vi "子界面-查看某框和报告生成-第2版-不显示界面.vi"(0 "框号":dbl format="%#_13g", 1 "框组":T3(array[cluster]), 3 "反射图原始路径":path, 5 "预先配置的灰度阈值":dbl, 6 "穿透图原始路径":path, 7 "部位信息":string[](array[string])=["", "34.500000", "32.500000", "1121", "34", "54.955926", "分层类", "不合格", ""], 12 "产品规格":cluster{"产品长度（周长）（mm）":dbl, "产品宽度（母线长）（mm）":dbl}) -> (14 "弥散类检测结果":string[][](table), 19 "分层类检测结果":string[][](table))   [LabVIEW 2018]
uses:
  <vilib>/vision/NI_Vision_Development_Module.lvlib
panel:
  out "弥散缺陷个数":i32
  out "分层缺陷个数":i32
  out "合格？ 弥散类":string="fencengThreshold"
  out "合格？分层类":string="fencengThreshold"
  out "?":T1(plugin-control)
  out "Threshold Image":T1(plugin-control)
  out "Threshold Image":T1(plugin-control)
  out "Threshold Image":T1(plugin-control)
  out "反射图ROI的最大灰度值":sgl
  in  "灰度阈值设置":cluster{"下限":dbl, "下限":dbl}(slide)={"下限"=0.0, "下限"=65.10638427734375} scale=0.0..255.0
  in  "Tab Control":T2
  out "穿透ROI":T1(plugin-control)
  out "Threshold Image":T1(plugin-control)
  out "?":T1(plugin-control)
  out "?":T1(plugin-control)
  out "Threshold Image":T1(plugin-control)
  out "Threshold Image":T1(plugin-control)
  out "弥散测量结果":dbl[][](array[numeric]) format="%.2f"
  in  "分隔符（'\\'代码显示）":string="\t"
  in  "格式字符串":string="%f"
  out "面积 (pixels)":i32
  in  "格式字符串 2":string="%f"
  in  "分隔符（'\\'代码显示）":string="\t"
  out "分层测量结果":dbl[][](array[numeric]) format="%.2f"
  out "缺陷分类的临界值":sgl format="%#.3f"
  # "所选区域信息"
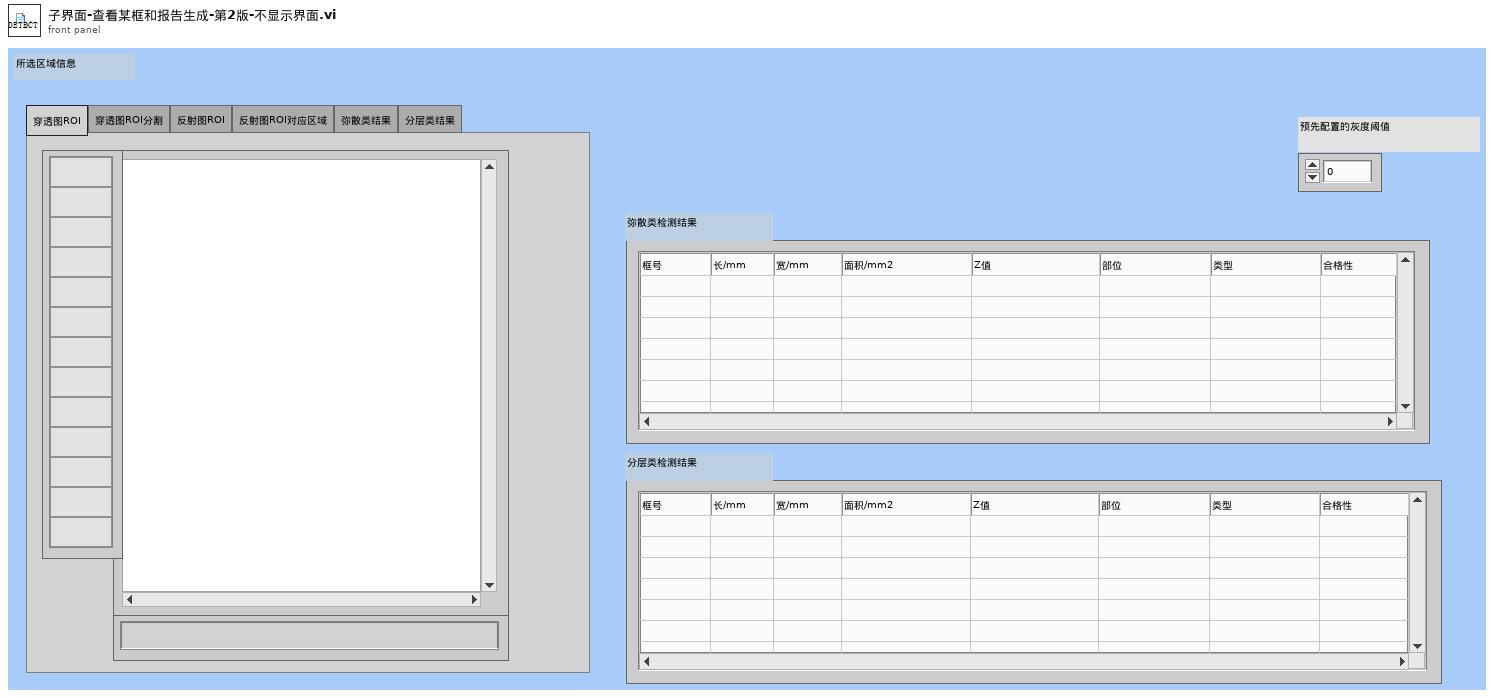
[diagram p1: front panel]
types:
  T1 = typedef "IMAQ Image.ctl" = refnum<image>
  T2 = typedef "控件 1.ctl" = enum32{"穿透图ROI", "穿透图ROI分割", "反射图ROI", "反射图ROI对应区域", "弥散类结果", "分层类结果"}
  T3 = cluster{"Global Rectangle":i32[], "Contours":cluster{"Contour Type":u32, "ROI Type":u32, "Points":i32[]}[]}[]
  T4 = typedef "Image Type" = u32
  T5 = typedef "Particle Parameters" = i32
  T6 = cluster{"Measurement Parameter":T5, "Range Lower Value":dbl, "Range Upper Value":dbl, "Range":bool, "Measurement Type":bool}[]
  T7 = cluster{"Global Rectangle":i32[], "Contours":cluster{"Contour Type":u32, "ROI Type":u32, "Points":i32[]}[]}
  T8 = cluster{"histogram":u32[], "Minimal Value":sgl, "Maximal Value":sgl, "Starting Value":sgl, "Interval Width":sgl, "Mean Value":sgl, "Standard  Variation":sgl, "Area (pixels)":i32}
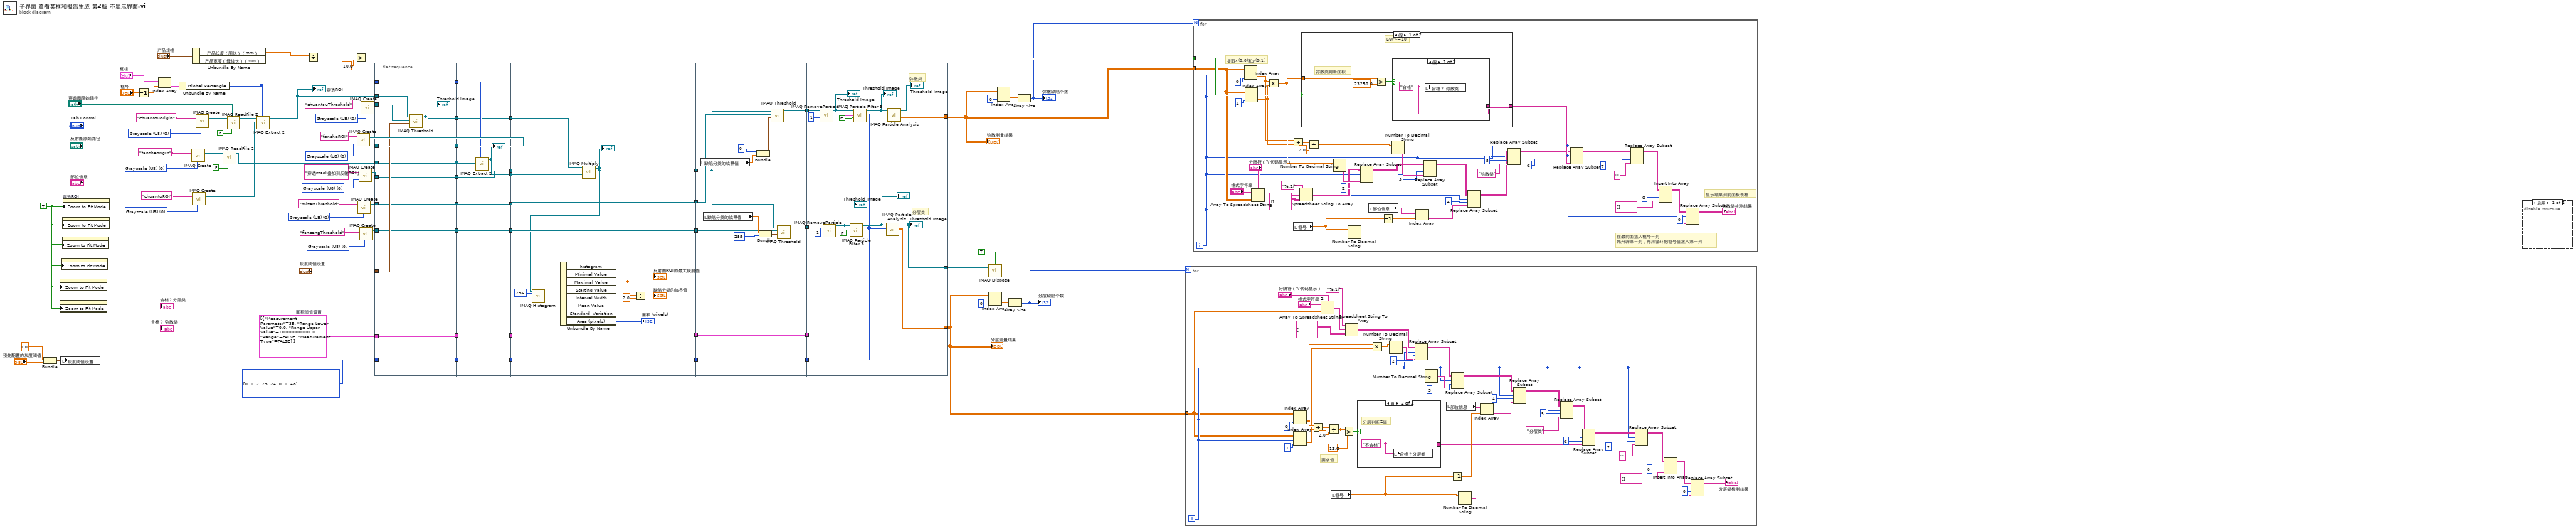
[diagram p0: block diagram]
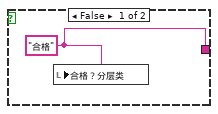
[diagram p2: hidden frame]
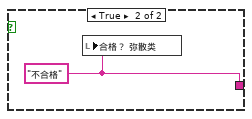
[diagram p3: hidden frame]
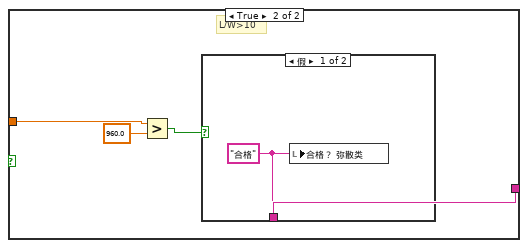
[diagram p4: hidden frame]
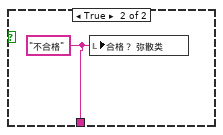
[diagram p5: hidden frame]
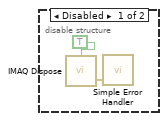
[diagram p6: hidden frame]
diagram:
  w48 = T4 0 items=["Grayscale (U8)", "Grayscale (I16)", "Grayscale (SGL)", "Complex (CSG)", "RGB (U32)", "HSL (U32)", "RGB (U64)", "Grayscale (U16)"] ("Image Type")
  w49 = T4 0 items=["Grayscale (U8)", "Grayscale (I16)", "Grayscale (SGL)", "Complex (CSG)", "RGB (U32)", "HSL (U32)", "RGB (U64)", "Grayscale (U16)"] ("Image Type")
  w50 = T4 0 items=["Grayscale (U8)", "Grayscale (I16)", "Grayscale (SGL)", "Complex (CSG)", "RGB (U32)", "HSL (U32)", "RGB (U64)", "Grayscale (U16)"] ("Image Type")
  w54 = T4 0 items=["Grayscale (U8)", "Grayscale (I16)", "Grayscale (SGL)", "Complex (CSG)", "RGB (U32)", "HSL (U32)", "RGB (U64)", "Grayscale (U16)"] ("Image Type")
  w58 = T4 0 items=["Grayscale (U8)", "Grayscale (I16)", "Grayscale (SGL)", "Complex (CSG)", "RGB (U32)", "HSL (U32)", "RGB (U64)", "Grayscale (U16)"] ("Image Type")
  w6 = i32[] [0, 1, 2, 23, 24, 0, 1, 48] items=["Bounding Rect Width", "Bounding Rect Height", "Area"] ("Pixel Measurements")
  w11 = T6 [{"Measurement Parameter"=35, "Range Lower Value"=0.0, "Range Upper Value"=10000000000.0, "Range"=FALSE, "Measurement Type"=FALSE}]  # 面积阈值设置
  w71 = T4 0 items=["Grayscale (U8)", "Grayscale (I16)", "Grayscale (SGL)", "Complex (CSG)", "RGB (U32)", "HSL (U32)", "RGB (U64)", "Grayscale (U16)"] ("Image Type")
  w41 = T4 0 items=["Grayscale (U8)", "Grayscale (I16)", "Grayscale (SGL)", "Complex (CSG)", "RGB (U32)", "HSL (U32)", "RGB (U64)", "Grayscale (U16)"] ("Image Type")
  w75 = T4 0 items=["Grayscale (U8)", "Grayscale (I16)", "Grayscale (SGL)", "Complex (CSG)", "RGB (U32)", "HSL (U32)", "RGB (U64)", "Grayscale (U16)"] ("Image Type")
  w84 = TRUE ("Zoom to Fit Mode")
  n1 = Bundle(0.0, "预先配置的灰度阈值"="预先配置的灰度阈值") -> (w82:cluster{dbl, "预先配置的灰度阈值":dbl})  [unwired: 1 in]
  n2 = property class="ImageControl"("Zoom to Fit Mode"=w84) -> ()  [unwired: 2 in, 2 out]
  n3 = property class="ImageControl"("Zoom to Fit Mode"=w84) -> ()  [unwired: 2 in, 2 out]
  n4 = local write "灰度阈值设置"(w82) -> ()
  n5 = property class="ImageControl"("Zoom to Fit Mode"=w84) -> ()  [unwired: 2 in, 2 out]
  n6 = property class="ImageControl"("Zoom to Fit Mode"=w84) -> ()  [unwired: 2 in, 2 out]
  n7 = property class="ImageControl"("Zoom to Fit Mode"=w84) -> ()  [unwired: 2 in, 2 out]
  n8 = property on="穿透ROI" class="ImageControl"("Zoom to Fit Mode"=w84) -> ()  [unwired: 2 in, 2 out]
  n9 = Decrement(x="框号") -> (x-1=w77:dbl)
  n10 = Index Array(array="框组", index=w77) -> (element=w78:T7)
  n11 = Unbundle By Name(w78) -> ("Global Rectangle"=w40:i32[])
  n12 = call "IMAQ Create"("Image Name"="fansheorigin", "Image Type"=w54) -> ("New Image"=w53:T1)  [unwired: 3 in, 1 out]
  n13 = call "IMAQ Create"("Image Name"="chuantuROI", "Image Type"=w58) -> ("New Image"=w57:T1)  [unwired: 3 in, 1 out]
  n14 = Unbundle By Name("产品规格") -> ("产品长度（周长）（mm）"=w66:dbl, "产品宽度（母线长）（mm）"=w65:dbl)
  n15 = call "IMAQ Create"("Image Name"="chuantouorigin", "Image Type"=w75) -> ("New Image"=w60:T1)  [unwired: 3 in, 1 out]
  n16 = call "IMAQ ReadFile 2"("Use File Path Image Type"=FALSE, "File Path"="反射图原始路径", "Image"=w53) -> ("Image Out"=w35:T1)  [unwired: 4 in, 4 out]
  n17 = call "IMAQ ReadFile 2"("Use File Path Image Type"=FALSE, "File Path"="穿透图原始路径", "Image"=w60) -> ("Image Out"=w61:T1)  [unwired: 4 in, 4 out]
  n18 = call "IMAQ Extract 2"("Optional Rectangle"=w40, "Image Dst"=w57, "Image Src"=w61) -> ("Image Dst Out"=w38:T1)  [unwired: 7 in, 1 out]
  "穿透ROI" <- w38
  n19 = Divide(x=w66, y=w65) -> (x/y=w69:dbl)
  n20 = Greater?(x=w69, y=10.0) -> (0:w64:bool)
  n21 = call "IMAQ Create"("Image Name"="fansheROI", "Image Type"=w41) -> ("New Image"=w36:T1)  [unwired: 3 in, 1 out]
  n22 = call "IMAQ Create"("Image Name"="misanThreshold", "Image Type"=w48) -> ("New Image"=w22:T1)  [unwired: 3 in, 1 out]
  n23 = call "IMAQ Create"("Image Name"="穿透mask叠加到反射ROI上", "Image Type"=w71) -> ("New Image"=w30:T1)  [unwired: 3 in, 1 out]
  n24 = call "IMAQ Create"("Image Name"="fencengThreshold", "Image Type"=w49) -> ("New Image"=w20:T1)  [unwired: 3 in, 1 out]
  n25 = call "IMAQ Create"("Image Name"="chuantouThreshold", "Image Type"=w50) -> ("New Image"=w39:T1)  [unwired: 3 in, 1 out]
  n26 = flat-sequence {
    tunnel: w40 -> [w96]
    tunnel: w39 -> [w95]
    tunnel: w38 -> [w94]
    tunnel: "灰度阈值设置" -> [w93]
    tunnel: w36 -> [w92]
    tunnel: w35 -> [w91]
    tunnel: [w96] -> w34
    tunnel: [w92] -> w33
    tunnel: [w91] -> w32
    tunnel: [w90] -> w31
    tunnel: w30 -> [w90]
    tunnel: [w89] -> w27
    tunnel: w22 -> [w88]
    tunnel: [w88] -> w24
    tunnel: [w87] -> w21
    tunnel: w20 -> [w87]
    tunnel: [w86] -> w12
    tunnel: w11 -> [w86]
    tunnel: [w85] -> w7
    tunnel: w6 -> [w85]
    tunnel: w34 -> [w106]
    tunnel: w33 -> [w104]
    tunnel: w32 -> [w105]
    tunnel: w31 -> [w103]
    tunnel: [w103] -> w29
    tunnel: [w102] -> w28
    tunnel: w27 -> [w102]
    tunnel: [w101] -> w26
    tunnel: w24 -> [w100]
    tunnel: [w100] -> w23
    tunnel: w21 -> [w99]
    tunnel: [w99] -> w19
    tunnel: w12 -> [w98]
    tunnel: [w98] -> w10
    tunnel: w7 -> [w97]
    tunnel: [w97] -> w5
    tunnel: w29 -> [w120]
    tunnel: w28 -> [w119]
    tunnel: w26 -> [w118]
    tunnel: [w117] -> w25
    tunnel: w23 -> [w117]
    tunnel: w19 -> [w116]
    tunnel: [w116] -> w18
    tunnel: [w109] -> w17
    tunnel: w10 -> [w108]
    tunnel: [w108] -> w9
    tunnel: w5 -> [w107]
    tunnel: [w107] -> w4
    tunnel: w25 -> [w128]
    tunnel: w18 -> [w127]
    tunnel: w17 -> [w126]
    tunnel: [w125] -> w14
    tunnel: [w124] -> w13
    tunnel: w9 -> [w123]
    tunnel: [w123] -> w8
    tunnel: w4 -> [w122]
    tunnel: [w122] -> w3
    tunnel: [w144] -> w16
    tunnel: [w139] -> w1
    tunnel: [w138] -> w15
    tunnel: w14 -> [w137]
    tunnel: w13 -> [w136]
    tunnel: w8 -> [w135]
    tunnel: w3 -> [w134]
    frame #0 {
      n27 = call "IMAQ Threshold"("Range"=w93, "Image Dst"=w95, "Image Src"=w94) -> ("Image Dst Out"=w89:T1)  [unwired: 3 in, 5 out]
      "Threshold Image" <- w89
    }
    frame #1 {
      n28 = call "IMAQ Extract 2"("Optional Rectangle"=w106, "Image Dst"=w105, "Image Src"=w104) -> ("Image Dst Out"=w101:T1)  [unwired: 7 in, 1 out]
      "?" <- w101
    }
    frame #2 {
      n29 = call "IMAQ Multiply"("Image Src A"=w119, "Image Dst"=w120, "Image Src B"=w118) -> ("Image Dst Out"=w109:T1)  [unwired: 4 in, 1 out]
      "?" <- w109
      n30 = call "IMAQ Histogram"("Number of Classes"=256, "Image"=w109) -> ("Histogram Report"=w112:T8)  [unwired: 8 in, 1 out]
      n31 = Unbundle By Name(w112) -> ("Maximal Value"=w114:sgl, "Area (pixels)"=→"面积 (pixels)":i32)  [unwired: 6 out]
      "反射图ROI的最大灰度值" <- w114
      n32 = Divide(x=w114, y=sgl 2.0) -> (x/y=→"缺陷分类的临界值":sgl)
    }
    frame #3 {
      n33 = local read "缺陷分类的临界值"() -> (w133:sgl)
      n34 = local read "缺陷分类的临界值"() -> (w131:sgl)
      n35 = Bundle(0, "缺陷分类的临界值"=w133) -> (w121:cluster{i32, "缺陷分类的临界值":sgl})  [unwired: 1 in]
      n36 = Bundle("缺陷分类的临界值"=w131, 255) -> (w130:cluster{"缺陷分类的临界值":sgl, i32})  [unwired: 1 in]
      n37 = call "IMAQ Threshold"("Range"=w121, "Image Dst"=w128, "Image Src"=w126) -> ("Image Dst Out"=w124:T1)  [unwired: 3 in, 5 out]
      n38 = call "IMAQ Threshold"("Range"=w130, "Image Dst"=w127, "Image Src"=w126) -> ("Image Dst Out"=w125:T1)  [unwired: 3 in, 5 out]
    }
    frame #4 {
      # "分层类"
      # "弥散类"
      n39 = call "IMAQ RemoveParticle"("Number of Erosion"=1, "Image Src"=w136) -> ("Image Dst Out"=w147:T1)  [unwired: 8 in, 1 out]
      "Threshold Image" <- w147
      n40 = call "IMAQ RemoveParticle"("Number of Erosion"=1, "Image Src"=w137) -> ("Image Dst Out"=w142:T1)  [unwired: 8 in, 1 out]
      "Threshold Image" <- w142
      n41 = call "IMAQ Particle Filter 3"("Image Src"=w142, "Keep/Remove Particles (F)"=FALSE) -> ("Image Dst Out"=w143:T1)  [unwired: 11 in, 2 out]
      "?" <- w143
      n42 = call "IMAQ Particle Filter 3"("Image Src"=w147, "Selection Values"=w135, "Keep/Remove Particles (F)"=FALSE) -> ("Image Dst Out"=w148:T1)  [unwired: 10 in, 2 out]
      "Threshold Image" <- w148
      n43 = call "IMAQ Particle Analysis"("Pixel Measurements"=w134, "Image"=w143) -> ("Particle Measurements (Pixels)"=w139:dbl[][], "Image Out (duplicate)"=w138:T1)  [unwired: 4 in, 4 out]
      "Threshold Image" <- w138
      n44 = call "IMAQ Particle Analysis"("Pixel Measurements"=w134, "Image"=w148) -> ("Particle Measurements (Real-World)"=w144:dbl[][], "Image Out (duplicate)"=→"Threshold Image":T1)  [unwired: 4 in, 4 out]
    }
  }
  n45 = call "IMAQ Dispose"("All Images? (No)"=TRUE, "Image"=w15) -> ()  [unwired: 4 in, 1 out]
  n46 = Index Array(array=w1, index (col)=0 ("禁用的索引 (列)")) -> (element=w46:dbl[])  [unwired: 1 in]
  n47 = Index Array(array=w16, index (col)=0 ("禁用的索引 (列)")) -> (element=w44:dbl[])  [unwired: 1 in]
  n48 = Array Size(array=w46) -> (size(s)=w2:i32)
  "分层缺陷个数" <- w2
  n49 = Array Size(array=w44) -> (size(s)=w63:i32)
  "弥散缺陷个数" <- w63
  n50 = for {
    N: w2 -> [_]
    tunnel: w1 -> [w150]
    i -> [w153]
    # "要求值"
    n51 = Index Array(array=w150, index (row)=w153, index (col)=0 ("禁用的索引 (列)")) -> (element=w167:dbl)
    n52 = Index Array(array=w150, index (row)=w153, index (col)=1 ("禁用的索引 (列)")) -> (element=w166:dbl)
    n53 = Add(x=w167, y=w166) -> (x+y=w193:dbl)
    n54 = Array To Spreadsheet String(delimiter (Tab)="分隔符（'\\'代码显示）", array=w150, 3:"格式字符串 2") -> (spreadsheet string=w192:string)
    n55 = Divide(x=w193, y=2.0) -> (x/y=w181:dbl)
    n56 = local read "框号"() -> (w151:dbl)
    n57 = Greater?(x=w181, y=13.0) -> (0:w194:bool)
    n58 = Spreadsheet String To Array(format string="%.1f", spreadsheet string=w192, array type (2D Dbl)=string[][] [] ("Array")) -> (array=w178:string[][])  [unwired: 1 in]
    n59 = case shown="真" w194 {
      tunnel: [w195 w196] -> w160
      frame False {
        w195 = "合格" ("合格？")
        n60 = local write "合格？分层类"(w195) -> ()
      }
      frame True {
        w196 = "不合格" ("合格？")
        # "分层判断Z值"
        n61 = local write "合格？分层类"(w196) -> ()
      }
    }
    n62 = Multiply(x=w167, y=w166) -> (x*y=w179:dbl)
    n63 = Number To Decimal String(number=w179) -> (decimal integer string=w165:string)  [unwired: 1 in]
    n64 = Replace Array Subset(array=w178, new element=w165, index (row)=w153, index (col)=2 ("禁用的索引 (列)")) -> (w174:string[][])
    n65 = Number To Decimal String(number=w181) -> (decimal integer string=w164:string)  [unwired: 1 in]
    n66 = local read "部位信息"() -> (w171:string[])
    n67 = Decrement(x=w151) -> (x-1=w170:dbl)
    n68 = Replace Array Subset(array=w174, new element=w164, index (row)=w153, index (col)=3 ("禁用的索引 (列)")) -> (w169:string[][])
    n69 = Number To Decimal String(number=w151) -> (decimal integer string=w152:string)  [unwired: 1 in]
    n70 = Index Array(array=w171, index=w170) -> (element=w163:string)
    n71 = Replace Array Subset(array=w169, new element=w163, index (row)=w153, index (col)=4 ("禁用的索引 (列)")) -> (w168:string[][])
    n72 = Replace Array Subset(array=w168, new element="分层类" ("新元素/子数组"), index (row)=w153, index (col)=5 ("禁用的索引 (列)")) -> (w173:string[][])
    n73 = Replace Array Subset(array=w173, new element=w160, index (row)=w153, index (col)=6 ("禁用的索引 (列)")) -> (w176:string[][])
    n74 = Replace Array Subset(array=w176, new element="" ("新元素/子数组"), index (row)=w153, index (col)=7 ("禁用的索引 (列)")) -> (w155:string[][])
    n75 = Insert Into Array(array=w155, index (col)=0 ("禁用的索引 (列)"), new element=string[] [] ("新元素/子数组")) -> (w157:string[][])  [unwired: 1 in]
    n76 = Replace Array Subset(array=w157, new element=w152, index (row)=w153, index (col)=0 ("禁用的索引 (列)")) -> (→"分层类检测结果":string[][])
  }
  n77 = for {
    N: w63 -> [_]
    tunnel: w64 -> [w240]
    tunnel: w16 -> [w239]
    i -> [w200]
    # "在最前面插入框号一列\n先开辟第一列，再用循环把框号值放入第一列"
    # "提取x(0,0)和y(0,1)"
    # "显示结果到前面板表格"
    n78 = Index Array(array=w239, index (row)=w200, index (col)=0 ("禁用的索引 (列)")) -> (element=w223:dbl)
    n79 = Index Array(array=w239, index (row)=w200, index (col)=1 ("禁用的索引 (列)")) -> (element=w222:dbl)
    n80 = Array To Spreadsheet String(delimiter (Tab)="分隔符（'\\'代码显示）", array=w239, 3:"格式字符串") -> (spreadsheet string=w237:string)
    n81 = Multiply(x=w223, y=w222) -> (x*y=w226:dbl)
    n82 = Add(x=w223, y=w222) -> (x+y=w225:dbl)
    n83 = local read "框号"() -> (w204:dbl)
    n84 = Spreadsheet String To Array(format string="%.1f", spreadsheet string=w237, array type (2D Dbl)=string[][] [] ("Array")) -> (array=w214:string[][])  [unwired: 1 in]
    n85 = case shown="假" w240 {
      tunnel: w226 -> [w243 w250]
      tunnel: [w241 w247] -> w238
      frame False {
        # "弥散类判断面积"
        # "L/W<=10"
        n86 = Greater?(x=w243, y=23250.0) -> (0:w242:bool)
        n87 = case shown="假" w242 {
          tunnel: [w245 w246] -> w241
          frame False {
            w245 = "合格" ("合格？")
            n88 = local write "合格？ 弥散类"(w245) -> ()
          }
          frame True {
            w246 = "不合格" ("合格？")
            n89 = local write "合格？ 弥散类"(w246) -> ()
          }
        }
      }
      frame True {
        # "L/W>10"
        n90 = Greater?(x=w250, y=960.0) -> (0:w248:bool)
        n91 = case shown="假" w248 {
          tunnel: [w251 w252] -> w247
          frame False {
            w251 = "合格" ("合格？")
            n92 = local write "合格？ 弥散类"(w251) -> ()
          }
          frame True {
            w252 = "不合格" ("合格？")
            n93 = local write "合格？ 弥散类"(w252) -> ()
          }
        }
      }
    }
    n94 = Divide(x=w225, y=2.0) -> (x/y=w219:dbl)
    n95 = Number To Decimal String(number=w226) -> (decimal integer string=w228:string)  [unwired: 1 in]
    n96 = Number To Decimal String(number=w204) -> (decimal integer string=w198:string)  [unwired: 1 in]
    n97 = Replace Array Subset(array=w214, new element=w228, index (row)=w200, index (col)=2 ("禁用的索引 (列)")) -> (w213:string[][])
    n98 = local read "部位信息"() -> (w209:string[])
    n99 = Decrement(x=w204) -> (x-1=w208:dbl)
    n100 = Number To Decimal String(number=w219) -> (decimal integer string=w221:string)  [unwired: 1 in]
    n101 = Index Array(array=w209, index=w208) -> (element=w207:string)
    n102 = Replace Array Subset(array=w213, new element=w221, index (row)=w200, index (col)=3 ("禁用的索引 (列)")) -> (w206:string[][])
    n103 = Replace Array Subset(array=w206, new element=w207, index (row)=w200, index (col)=4 ("禁用的索引 (列)")) -> (w205:string[][])
    n104 = Replace Array Subset(array=w205, new element="弥散类" ("新元素/子数组"), index (row)=w200, index (col)=5 ("禁用的索引 (列)")) -> (w212:string[][])
    n105 = Replace Array Subset(array=w212, new element=w238, index (row)=w200, index (col)=6 ("禁用的索引 (列)")) -> (w211:string[][])
    n106 = Replace Array Subset(array=w211, new element="" ("新元素/子数组"), index (row)=w200, index (col)=7 ("禁用的索引 (列)")) -> (w203:string[][])
    n107 = Insert Into Array(array=w203, index (col)=0 ("禁用的索引 (列)"), new element=string[] [] ("新元素/子数组")) -> (w201:string[][])  [unwired: 1 in]
    n108 = Replace Array Subset(array=w201, new element=w198, index (row)=w200, index (col)=0 ("禁用的索引 (列)")) -> (→"弥散类检测结果":string[][])
  }
  n109 = disable-structure shown="启用" {
    frame Disabled {
      n110 = call "IMAQ Dispose"("All Images? (No)"=TRUE) -> ("error out"=w254:errorcluster)  [unwired: 5 in]
      n111 = call <vilib>:"Simple Error Handler.vi"("error in (no error)"=w254) -> ()  [unwired: 4 in, 5 out]
    }
    frame Enabled {
    }
  }
  "分层测量结果" <- w1
  "弥散测量结果" <- w16
